vi "Build Script Error Template.vi"(8 "error in (no error)":errorcluster, 9 "String to Append":string, 10 "Error":T1, 11 "Insert Error":bool=TRUE) -> (0 "error out":errorcluster)   [LabVIEW 2021, in "Build Script Common.lvlib" / "Errors_CIF_U.lvlib"]
uses:
  <vilib>/CIF Foundation/CIF Utilities/Errors/Errors_CIF_U.lvlib
  Typedef/Build Script Errors.ctl
  Build Script Common.lvlib
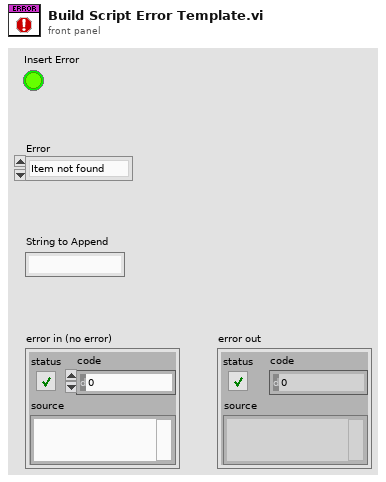
[diagram p1: front panel]
types:
  T1 = typedef "Build Script Common.lvlib/Build Script Errors.ctl" = enum16{"Item not found"}
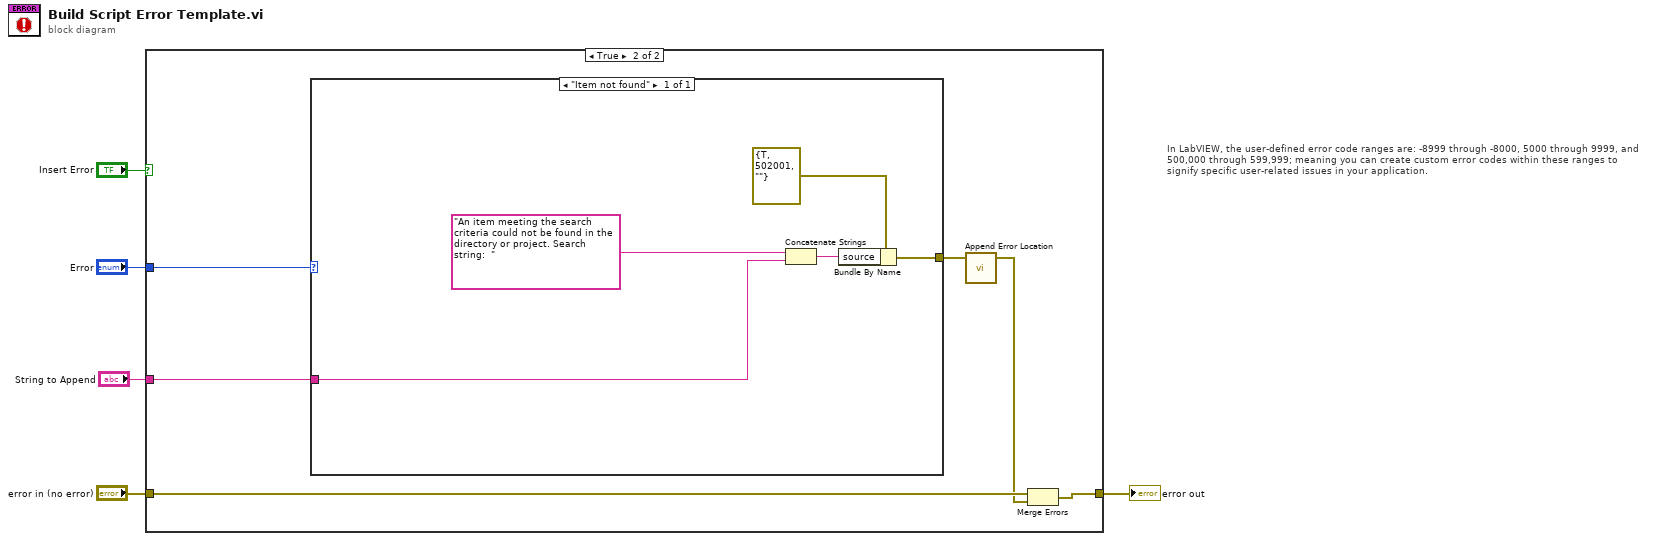
[diagram p0: block diagram]
diagram:
  # "In LabVIEW, the user-defined error code ranges are: -8999 through -8000, 5000 through 9999, and 500,000 through 599,999; meaning you can create custom error codes within these ranges to signify specific user-related issues in your application."
  n1 = case shown="True" "Insert Error" {
    tunnel: [w6 w9] -> w4
    tunnel: "error in (no error)" -> [w6 w10]
    tunnel: "Error" -> [_ w12]
    tunnel: "String to Append" -> [_ w11]
    frame False {
    }
    frame True {
      n2 = case shown="\"Item not found\"" w12 {
        tunnel: w11 -> [w14]
        tunnel: [w16] -> w8
        frame "Item not found" {
          n3 = Concatenate Strings("An item meeting the search criteria could not be found in the directory or project. Search string:  " ("source"), w14) -> (w13:string)
          n4 = Bundle By Name(cluster=errorcluster {"status"=TRUE, "code"=502001, "source"=""} ("Invalid ID"), "source"=w13) -> (w16:errorcluster)
        }
      }
      n5 = call <vilib>:"Append Error Location.vi"("error in (no error)"=w8) -> ("error out"=w7:errorcluster)  [unwired: 4 in]
      n6 = Merge Errors(w10, w7) -> (w9:errorcluster)
    }
  }
  "error out" <- w4
